vi "Write Multiple IO Card.vi"(5 "parity (0:none)":enum16{"None", "Odd", "Even", "Mark", "Space"}(ring), 7 "Check Info":string="OK", 8 "error in (no error)":errorcluster, 9 "write buffer":string[](array[string]), 10 "baud rate (9600)":u32=1000000, 11 "VISA resource name":refnum<visa-resource-name>) -> (0 "error out":errorcluster, 2 "read buffer":string[](array[string]), 3 "VISA resource name out":refnum<visa-resource-name>)   [LabVIEW 2020]
uses:
  e74a2754-96b5-4d25-ac7b-846f49a606ad.vi
  <vilib>/Instr/_visa.llb/VISA Configure Serial Port (Instr).vi
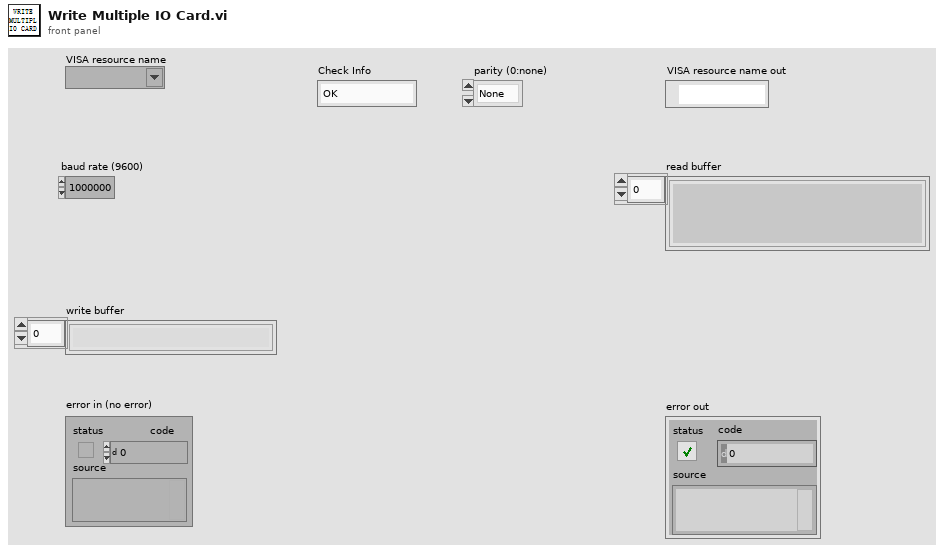
[diagram p1: front panel]
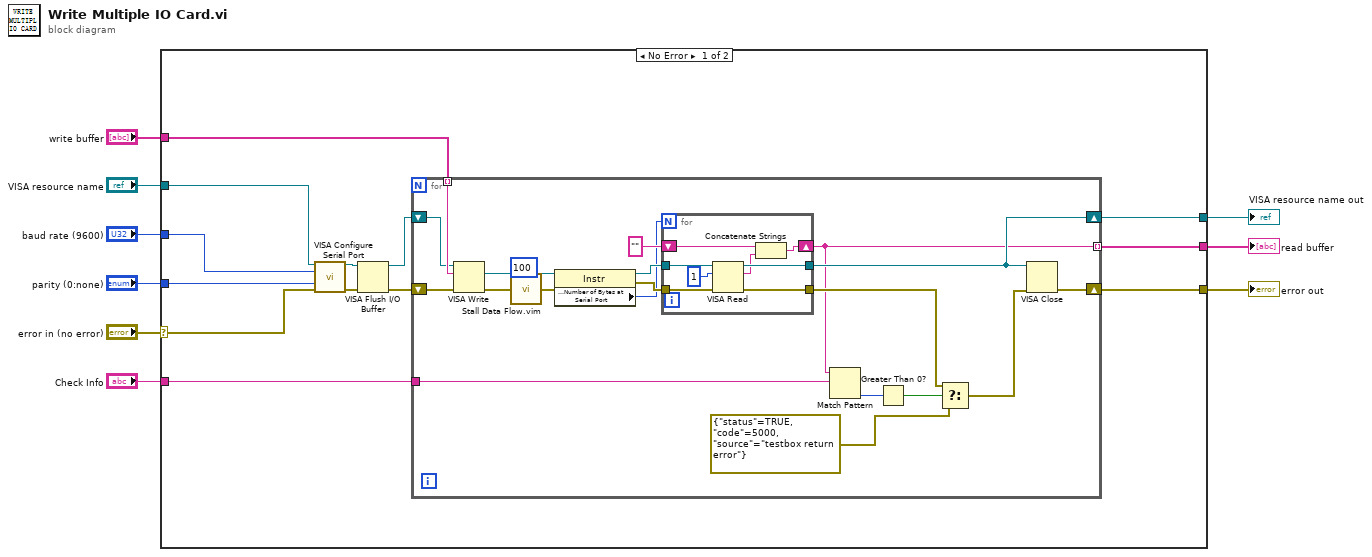
[diagram p0: block diagram]
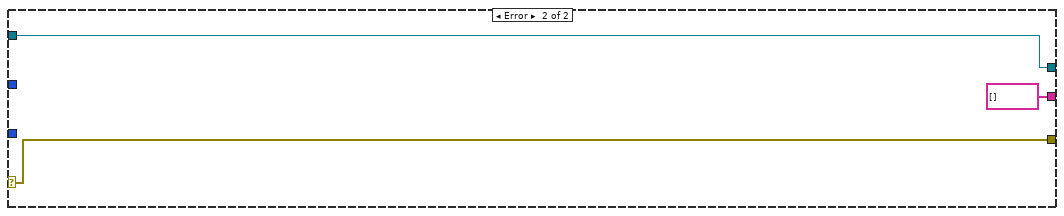
[diagram p2: hidden frame]
diagram:
  n1 = case shown="No Error" "error in (no error)" {
    selector: "error in (no error)" -> [w16 w53]
    tunnel: [w22 w53] -> w9
    tunnel: "VISA resource name" -> [w21 w52]
    tunnel: "parity (0:none)" -> [w20 _]
    tunnel: "baud rate (9600)" -> [w19 _]
    tunnel: "write buffer" -> [w18 _]
    tunnel: "Check Info" -> [w17 _]
    tunnel: [w15 w52] -> w2
    tunnel: [w10 string[] []] -> w1
    frame No Error {
      n2 = call-poly "VISA Configure Serial Port"("VISA resource name"=w21, "baud rate (9600)"=w19, "parity (0:none)"=w20, "error in (no error)"=w16) -> ("VISA resource name out"=w13:refnum<visa-resource-name>, "error out"=w14:errorcluster)  [unwired: 10 in]
      n3 = VISA Flush I/O Buffer(VISA resource name=w13, error in (no error)=w14) -> (VISA resource name out=w12:refnum<visa-resource-name>, error out=w11:errorcluster)  [unwired: 1 in]
      n4 = for {
        tunnel: w18 -> [w41] mode=indexing
        tunnel: w17 -> [w40]
        shift-right: [w39] -> w15
        shift-left: w12 -> [w35]
        shift-right: [w42] -> w22
        shift-left: w11 -> [w34]
        tunnel: [w23] -> w10 mode=indexing
        n5 = VISA Write(VISA resource name=w35, write buffer=w41, error in (no error)=w34) -> (VISA resource name out=w33:refnum<visa-resource-name>, error out=w38:errorcluster)  [unwired: 1 out]
        n6 = call "Stall Data Flow.vim"("value in"=w38, "milliseconds to wait"=u32 100) -> ("value out"=w31:errorcluster)  [unwired: 1 out]
        n7 = property class="Instr"(reference=w33, error in=w31) -> (reference out=w32:refnum<visa-resource-name>, error out=w30:errorcluster, "Serial Settings:Number of Bytes at Serial Port"=w29:u32)
        n8 = for {
          N: w29 -> [_]
          shift-right: [w47] -> w23
          shift-left: "" -> [w48]
          tunnel: w32 -> [w46]
          tunnel: [w50] -> w39
          tunnel: w30 -> [w45]
          tunnel: [w49] -> w24
          n9 = VISA Read(VISA resource name=w46, byte count=u32 1, error in (no error)=w45) -> (VISA resource name out=w50:refnum<visa-resource-name>, read buffer=w43:string, error out=w49:errorcluster)  [unwired: 1 out]
          n10 = Concatenate Strings(w48, w43) -> (w47:string)
        }
        n11 = Match Pattern(string=w23, regular expression=w40) -> (offset past match=w28:i32)  [unwired: 1 in, 3 out]
        n12 = Greater Than 0?(x=w28) -> (x > 0?=w27:bool)
        n13 = Select(t=w24, s=w27, f=errorcluster {"status"=TRUE, "code"=5000, "source"="testbox return error"}) -> (s? t:f=w25:errorcluster)
        n14 = VISA Close(VISA resource name=w39, error in (no error)=w25) -> (error out=w42:errorcluster)
      }
    }
    frame Error {
    }
  }
  "error out" <- w9
  "read buffer" <- w1
  "VISA resource name out" <- w2
